vi "DataSimulateModule.vi"(7 "Name(\"\" to use uuid)":string="JKISM-Module") -> ()   [LabVIEW 2014]
uses:
  <userlib>/_NEVSTOP/JKI State Machine++/_Polymophic/Add State(s) to Queue By BOOL(Element).vi
  <userlib>/_NEVSTOP/JKI State Machine++/_Support/JKISMQ/_Obtain JKISMQ.vi
  <userlib>/_NEVSTOP/JKI State Machine++/_Support/FGV-BroadcastRegistry/Cache-Broadcast Registry Search Result.vi
  <userlib>/_NEVSTOP/JKI State Machine++/_Support/JKISMQ/_Create Resp Queue.vi
  <userlib>/_NEVSTOP/JKI State Machine++/_Support/JKISMQ/_Unlock JKISMQ.vi
  <userlib>/_NEVSTOP/JKI State Machine++/_Support/JKISMQ/_Lock State JKISMQ.vi
  <userlib>/_NEVSTOP/JKI State Machine++/_Support/JKISMQ/_Release JKISMQ.vi
  <userlib>/_NEVSTOP/JKI State Machine++/_Support/JKISMQ/_Input Name to JKISM Mode.vi
  <userlib>/_NEVSTOP/JKI State Machine++/Utility/uuid.vi
  <userlib>/_NEVSTOP/JKI State Machine++/_Support/FGV-BroadcastRegistry/global-JKISMQ FGV Change Flag.vi
  <userlib>/_NEVSTOP/JKI State Machine++/_Support/JKISMQ/_JKISMQFGV.vi
  <userlib>/_NEVSTOP/JKI State Machine++/_Support/GlobalEvent/FGV-GlobalEventRef.vi
  <userlib>/_NEVSTOP/JKI State Machine++/_Support/JKISMQ/_Dequeue JKISMQ.vi
  <userlib>/_NEVSTOP/JKI State Machine++/_Support/JKISMQ/_Enqueue JKISMQ.vi
  <userlib>/_NEVSTOP/JKI State Machine++/_Support/FGV-BroadcastRegistry/global-Broadcast Cache Change Flag.vi
  <userlib>/_NEVSTOP/JKI State Machine++/_Support/FGV-BroadcastRegistry/FGV-BroadcastRegistry.vi
  Array-Parameter/_support/FGV-MassData.vi
  Array-Parameter/JKISM++ Array Parameter Support.lvlib
panel:
  out "Error Occurred":errorcluster
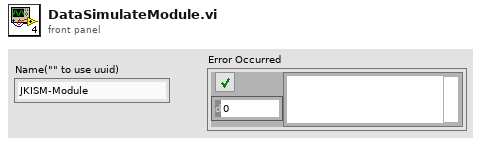
[diagram p1: front panel]
types:
  T1 = enum32{"Invalid", "Standard", "Closed", "Hidden", "Minimized", "Maximized"}
  T2 = enum32{"invalid app kind", "Development System", "Run Time System", "Student Edition", "Embedded LabVIEW", "Evaluation", "Custom"}
  T3 = cluster{"Core":cluster{"Current VI Reference":refnum<vi>, "Close Panel on Exit?":bool}, "DataGen?":bool, "DataSize":i32}
  T4 = cluster{"Current VI Reference":refnum<vi>, "Close Panel on Exit?":bool}
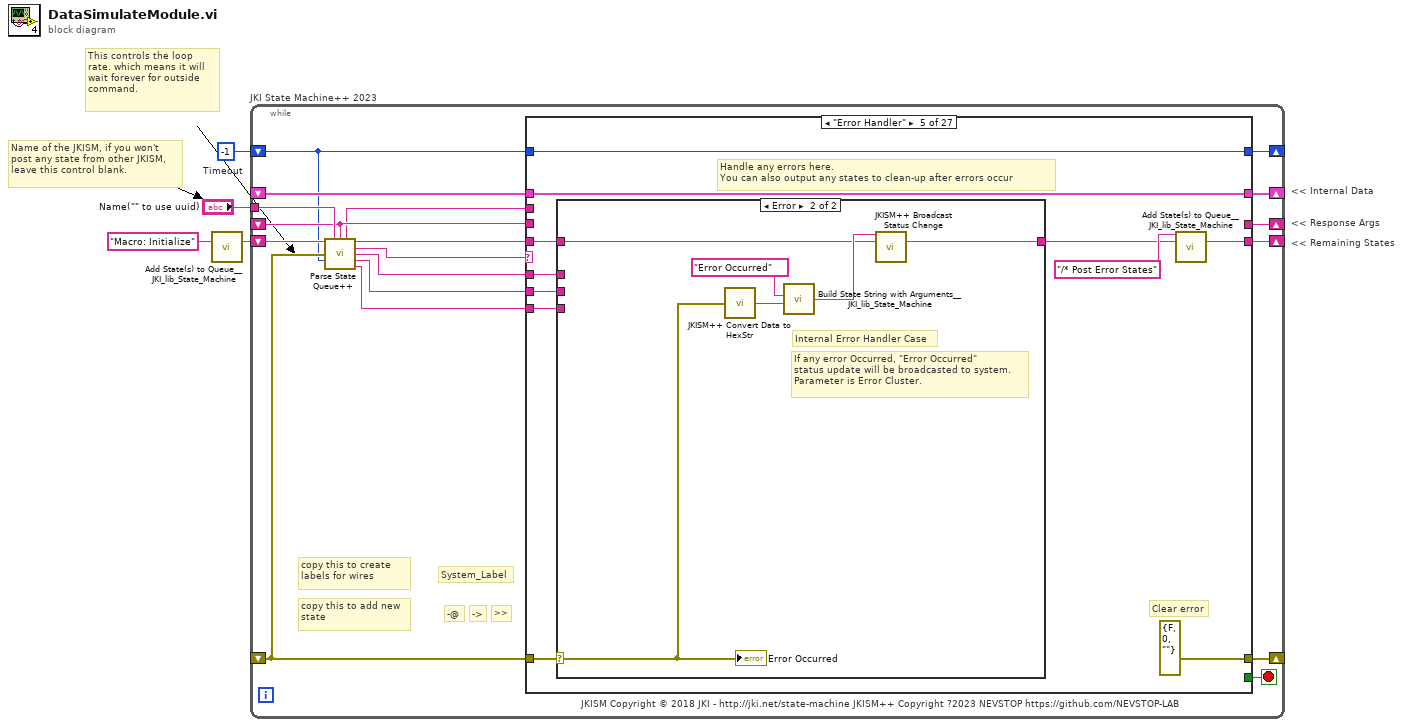
[diagram p0: block diagram]
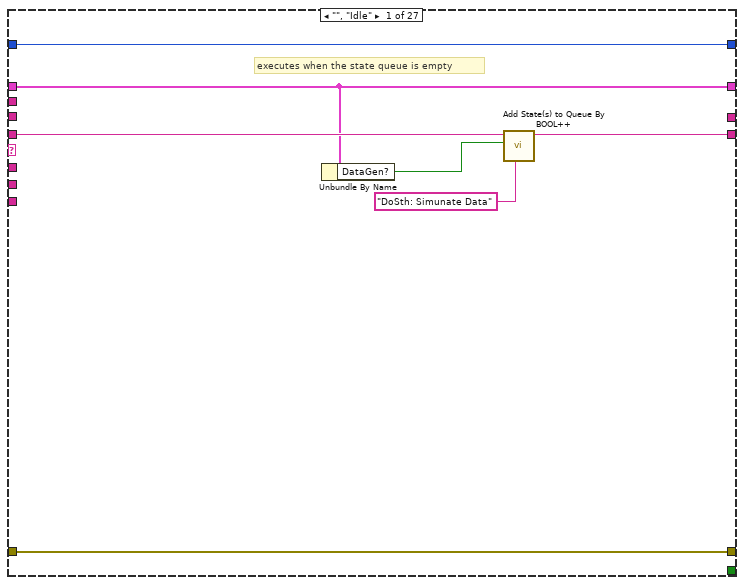
[diagram p2: hidden frame]
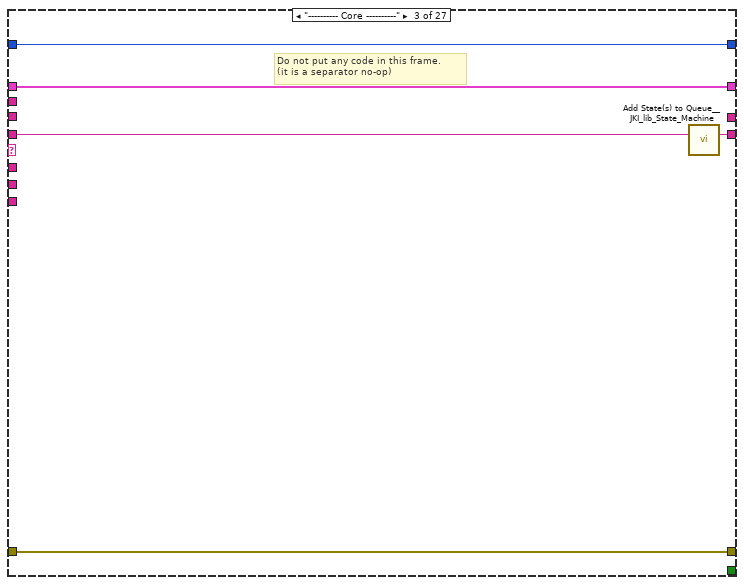
[diagram p4: hidden frame]
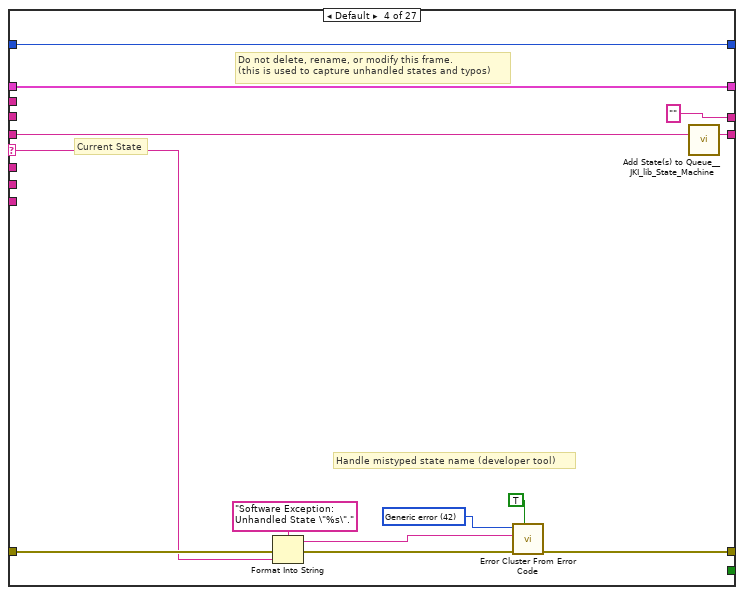
[diagram p5: hidden frame]
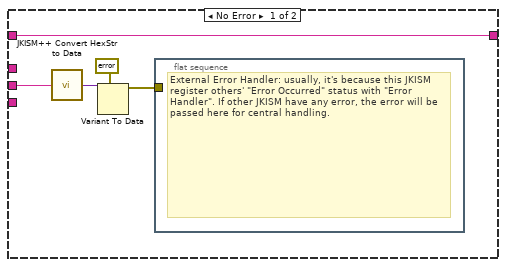
[diagram p6: hidden frame]
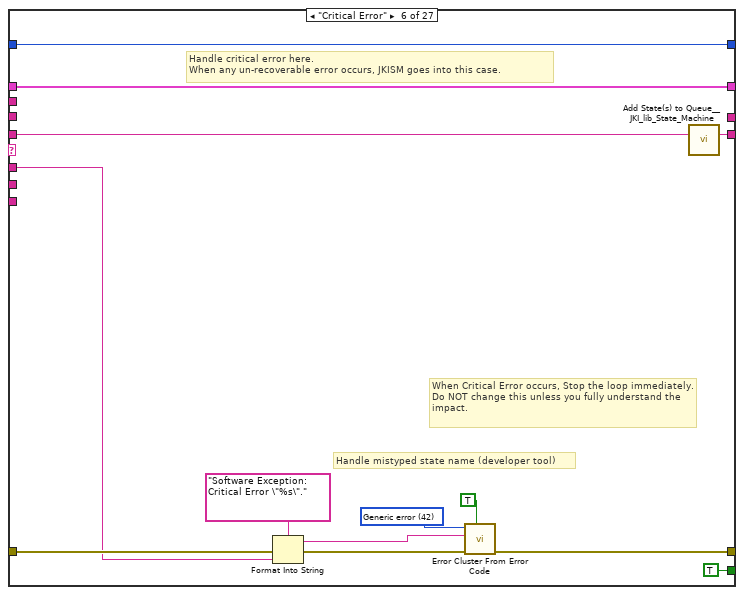
[diagram p7: hidden frame]
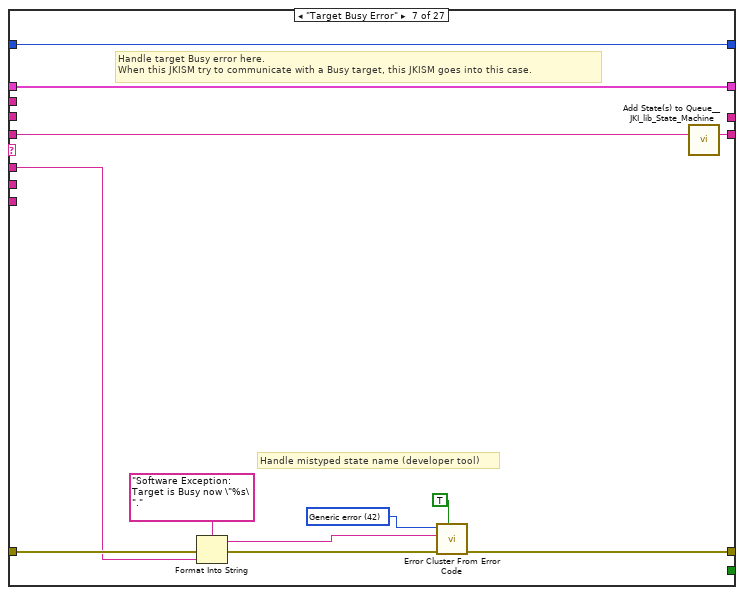
[diagram p8: hidden frame]
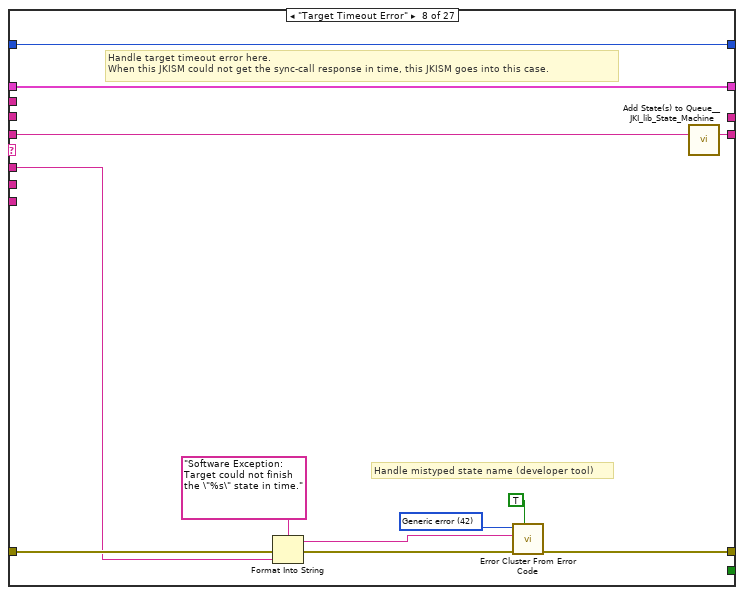
[diagram p9: hidden frame]
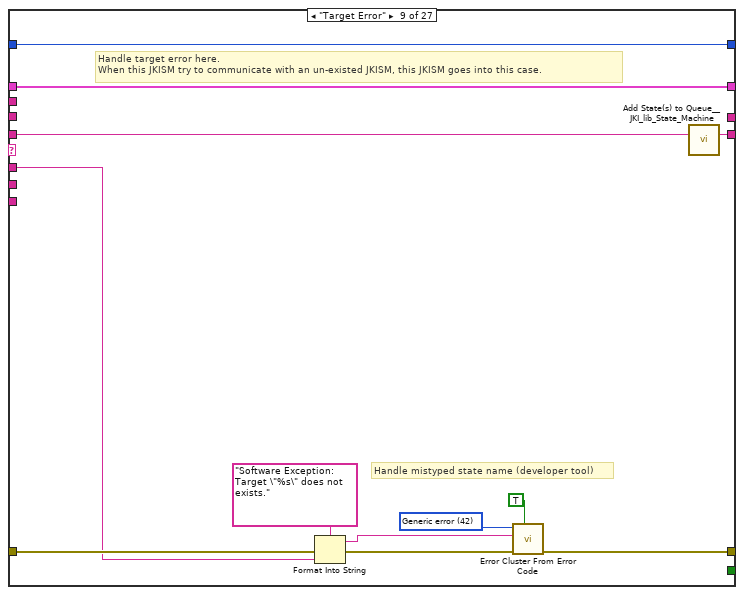
[diagram p10: hidden frame]
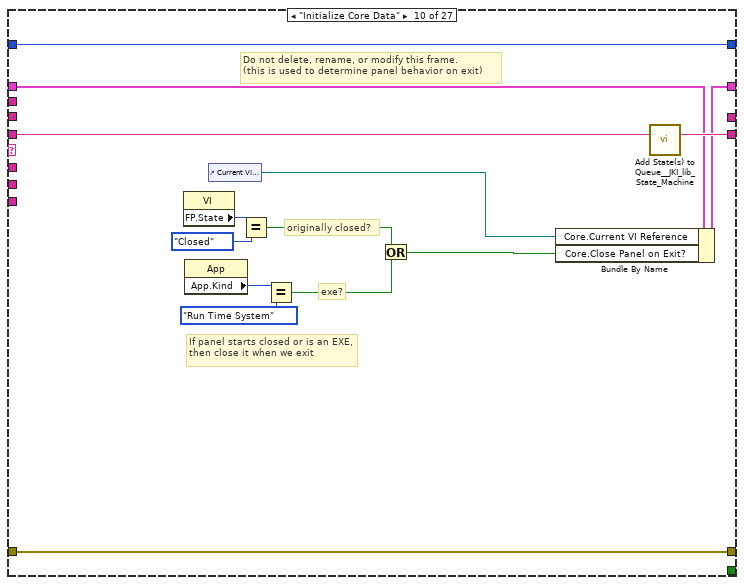
[diagram p11: hidden frame]
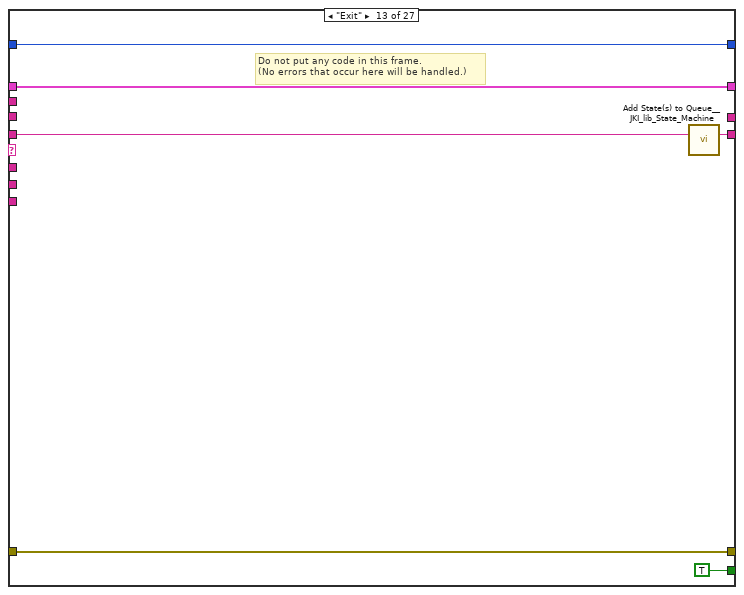
[diagram p14: hidden frame]
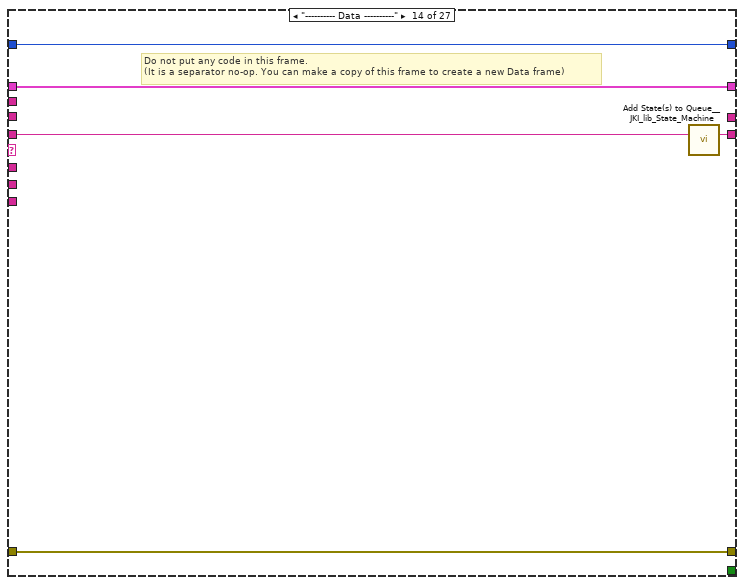
[diagram p15: hidden frame]
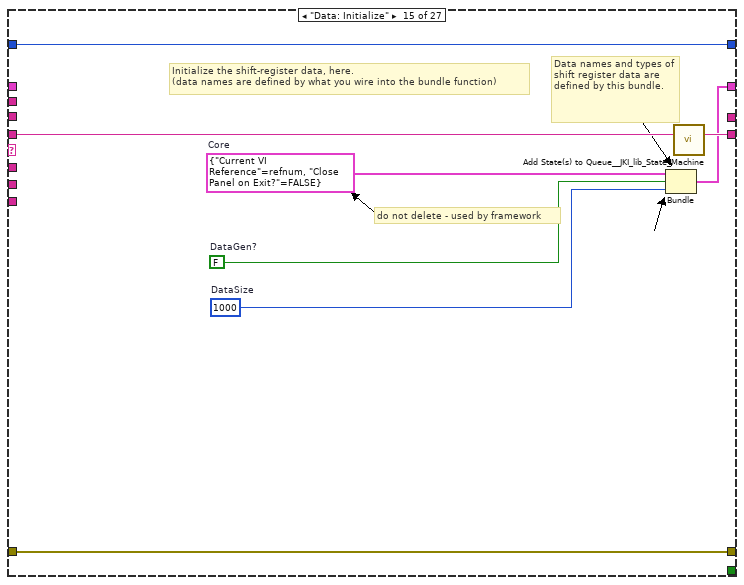
[diagram p16: hidden frame]
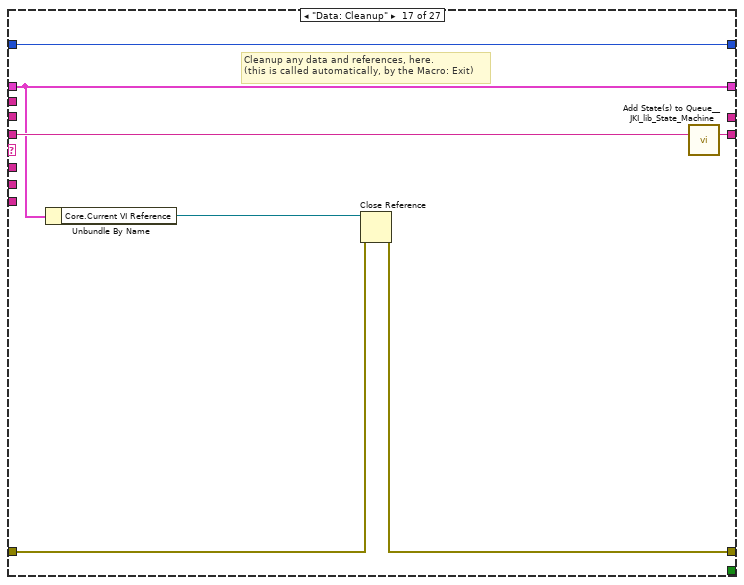
[diagram p18: hidden frame]
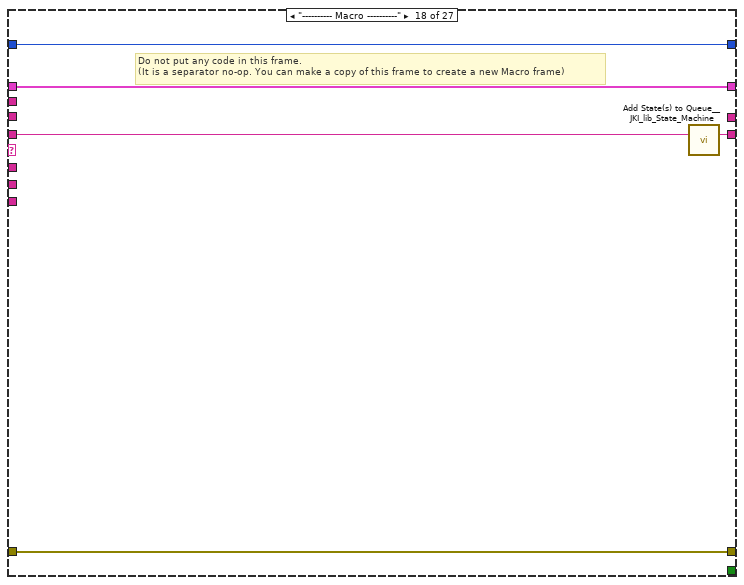
[diagram p19: hidden frame]
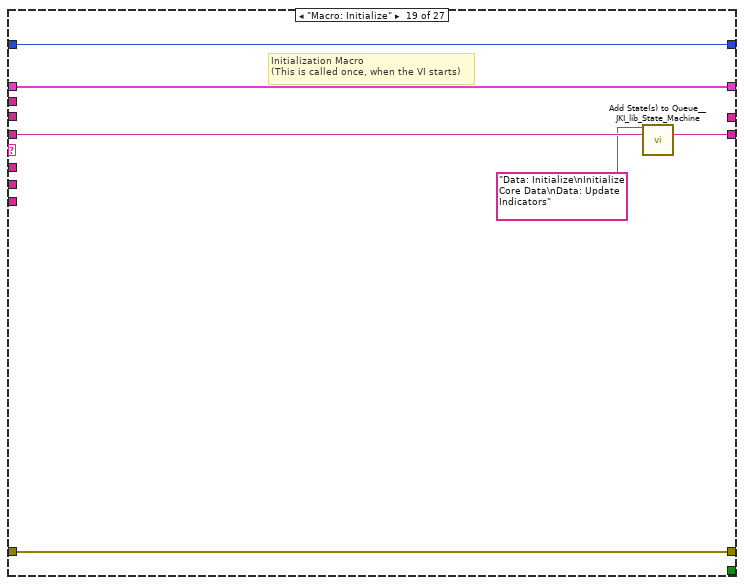
[diagram p20: hidden frame]
diagram:
  w1 = -1  # Timeout
  # "<< Internal Data"
  # "<< Response Args"
  # "<< Remaining States"
  # "Name of the JKISM, if you won't post any state from other JKISM,  leave this control blank."
  # "This controls the loop rate. which means it will wait forever for outside  command."
  n1 = call <vilib>:"Add State(s) to Queue__JKI_lib_State_Machine.vi"("State(s) in (\"\")"="Macro: Initialize") -> ("States Out"=w2:string)  [unwired: 14 in]
  n2 = while "JKI State Machine++ 2023" {
    shift-right: [w17] -> _
    shift-left: _ -> [w16]
    shift-right: [w20] -> _
    shift-left: _ -> [w15]
    shift-right: [w19] -> _
    shift-left: w2 -> [w21]
    tunnel: "Name(\"\" to use uuid)" -> [w13]
    shift-right: [w14] -> _
    shift-left: _ -> [w8]
    shift-right: [w6] -> _
    shift-left: w1 -> [w5]
    stop <- w18 stop-if-true
    # "JKISM Copyright © 2018 JKI - http://jki.net/state-machine JKISM++ Copyright ?2023 NEVSTOP https://github.com/NEVSTOP-LAB"
    # ">>"
    # "copy this to add new state"
    # "->"
    # "-@"
    # "copy this to create labels for wires"
    # "System_Label"
    n3 = call <userlib>:"Parse State Queue++.vi"("State Queue"=w21, "Name(\"\" to use uuid)"=w13, "Response Arguments"=w8, "Error In (no error)"=w15, "Dequeue Timeout(0ms)"=w5) -> ("Name Used"=w7:string, "Remaining States"=w22:string, "Current State"=w9:string, "Arguments"=w10:string, "Argument - State"=w11:string, "From Who"=w12:string)  [unwired: 5 in]
    n4 = case shown="\"Error Handler\"" w9 {
      selector: w9 -> [_ _ _ w41 _ _ _ _ _ _ _ _ _ _ _ _ _ _ _ _ _ _ _ _ _ _ _]
      tunnel: w22 -> [w27 w32 w38 w45 w56 w80 w93 w105 w117 w136 w139 w143 w150 w155 w163 w166 w174 w179 w185 w191 w194 w200 w207 w213 w219 w225 w238]
      tunnel: w10 -> [_ _ _ _ w55 w76 w89 w101 w113 _ _ _ _ _ _ _ _ _ _ _ _ _ w203 _ _ _ _]
      tunnel: w16 -> [w26 w31 w35 w43 w61 w78 w91 w103 w115 w129 w138 w142 w148 w152 _ w165 w169 w176 w182 w188 w193 w199 w206 w212 w218 w222 w232]
      tunnel: [w29 w33 w36 w47 errorcluster {"status"=FALSE, "code"=0, "source"=""} ("error out") w82 w88 w100 w112 w133 w140 w144 w147 w153 w160 w167 w170 w177 w183 w189 w195 w201 w208 w214 w220 w223 w236] -> w20
      tunnel: w15 -> [w29 w33 w36 w46 w59 w81 w94 w106 w118 w133 w140 w144 w147 w153 w160 w167 w171 w177 w183 w189 w195 w201 w208 w214 w220 w223 w236]
      tunnel: [w28 w32 w37 w44 w57 w79 w92 w104 w116 w135 w139 w143 w149 w154 w162 w166 w173 w178 w184 w190 w194 w200 w207 w213 w219 w224 w237] -> w19
      tunnel: [_ _ _ _ _ TRUE _ _ _ _ _ _ TRUE _ _ _ _ _ _ _ _ _ _ _ _ _ _] -> w18
      tunnel: [w26 w31 w35 w43 w61 w78 w91 w103 w115 w134 w138 w142 w148 w152 w161 w165 w169 w176 w182 w188 w193 w198 w205 w212 w217 w222 w232] -> w17
      tunnel: w12 -> [_ _ _ _ w54 _ _ _ _ _ _ _ _ _ _ _ _ _ _ _ _ _ _ _ _ _ _]
      tunnel: w11 -> [_ _ _ _ w53 _ _ _ _ _ _ _ _ _ _ _ _ _ _ _ _ _ _ _ _ _ _]
      tunnel: [_ _ _ "" _ _ _ _ _ _ _ _ _ _ _ _ _ _ _ _ _ _ _ w210 _ _ _] -> w14
      tunnel: w7 -> [_ _ _ _ _ _ _ _ _ _ _ _ _ _ _ _ _ _ _ _ _ _ _ _ _ _ _]
      tunnel: w8 -> [_ _ _ _ _ _ _ _ _ _ _ _ _ _ _ _ _ _ _ _ _ _ _ _ _ _ _]
      tunnel: [w23 w30 w34 w39 w52 w74 w87 w99 w111 w123 w137 w141 w145 w151 w156 w164 w168 w175 w180 w186 w192 200 ("Timeout") w202 w209 -1 ("Timeout") w221 w229] -> w6
      tunnel: w5 -> [w23 w30 w34 w39 w52 w74 w87 w99 w111 w123 w137 w141 w145 w151 w156 w164 w168 w175 w180 w186 w192 _ w202 w209 _ w221 w229]
      frame "", "Idle" {
        # "executes when the state queue is empty"
        n5 = Unbundle By Name(w26) -> ("DataGen?"=w25:bool)
        n6 = call-poly <userlib>:"Add State(s) to Queue By BOOL++.vi"("TRUE(\"\")"="DoSth: Simunate Data" ("TRUE(\"\")"), "Bool"=w25, "State Queue(\"\")"=w27) -> ("State Queue Out"=w28:string)  [unwired: 8 in]
      }
      frame "JKISM++ Documentation" {
        # "JKISM++ Documentation"
        # "State Syntax:\nStateCategory: State >> Argument -@ JKISMName\nStateCategory: State >> Argument -> JKISMName\n\nLine Terminator: Line feed"
        # "Commenting:\nTo add a comment use \"//\" or \"#\" and all text to the right will be ignored\nCommenting Example:\nUI: Initialize // This initializes the UI\n// Another comment line"
        # "Example:\nUI: Help >> About -@Main\nUI: Help >> About ->Main\n\nWhere \"UI\" is the state category\nWhere \"Help\" is the state\nWhere \"About\" is the argument\nWhere \"Main\" is the Name of JKISM,which actually run the \"UI: Help >> About\"\n\n    \"-@\" stands for sync state. Current JKISM will wait until the state is finished. \n            - if \"Main\" named JKISM does not exist, \"Target Error\" will occur.\n            - if \"Main\" named JKISM is in another sync remote state, \"Target Busy Error\" will occur.\n            - if \"Main\" named JKISM could not finish the state in time, \"Target Timeout Error\" will occur.\n            - if everything is right. \"Response\" will occur with Argument back from \"Main\" named JKISM. \n\n    \"->\" stands for async state. Current JKISM will post the state and continue to next state in next iteration.\n            - if \"Main\" named JKISM does not exist, \"Target Error\" will occur.\n            - if everything is right. \"Async Message Posted\" will occur.\n            - After State is finished. Caller will receive a \"Async Response\" state from callee.\n\nWhen duplicated name is used for multiple JKISM module or some framework problem happens, \"Critical Error\" will occur."
      }
      frame "---------- Core ----------" {
        # "Do not put any code in this frame.\n(it is a separator no-op)"
        n7 = call <vilib>:"Add State(s) to Queue__JKI_lib_State_Machine.vi"("State(s) in (\"\")"=w38) -> ("States Out"=w37:string)  [unwired: 14 in]
      }
      frame Default {
        w50 = 42 items=["No error", "Argument error", "Memory is full", "Out of zone", "End of file", "File already open", "Generic file I/O error", "File not found", "File permission error", "Disk is full", "Duplicate path", "Too many files open", "System feature not enabled", "Resource file not found", "Cannot add resource", "Resource not found", "Image not found", "Image memory error", "Pen does not exist", "Config type invalid", "Config token not found", "Config parse error", "Config memory error", "Bad external code format", "Bad external code offset", "External code not present", "Null window", "Destroy window error", "Null menu", "Print aborted", "Bad print record", "Print driver error", "Windows error during printing", "Memory error during printing", "Print dialog error", "Generic print error", "Invalid device refnum", "Device not found", "Device parameter error", "Device unit error", "Cannot open device", "Device call aborted", "Generic error", "Cancelled by user", "Object ID too low", "Object ID too high", "Object not in heap", "Unknown heap", "Unknown object (invalid DefProc)", "Unknown object (DefProc not in table)", "Message out of range", "Invalid (null) method", "Unknown message", "Manager call not supported", "Bad address", "Network operation in progress", "Network operation timed out", "Connection is busy", "Network attribute not supported", "Network error", "Address in use", "System out of memory", "Connection aborted", "Connection refused", "Not connected", "Already connected", "Connection closed", "Initialization error (interapplication manager)", "Bad occurrence", "Wait on unbound occurrence handler", "Occurrence queue overflow", "Datalog type conflict", "Unused", "Unrecognized type (interapplication manager)", "Memory corrupt", "Failed to make temporary DLL", "Old CIN version", "Drag socket not found", "Failed to load drop-object", "Failed to register OLE object", "Failed to release OLE object", "Format specifier type mismatch", "Unknown format specifier", "Too few format specifiers", "Too many format specifiers", "Scan failed", "Newer CIN version", "Error converting to variant", "Runtime menu error", "Password tampered", "Variant attribute not found", "Incompatible variant data type", "Event data is not available", "Event Store is not present", "Occurrence is not found", "Event Queue is not created", "Event info is not available", "Refnum passed is NULL", "Error retrieving Class GUID", "Error retrieving CoClass GUID", "Error retrieving TypeLib GUID.", "Bad built application magic bytes.", "Specific driver is different from the specific driver associated with the Logical Name.", "There is no session opened to the class driver.", "Max Error", "MAX - Error with config objects", "MAX - Error loading configuration", "MAX - Group not supported"]
        # "Current State"
        # "Do not delete, rename, or modify this frame.\n(this is used to capture unhandled states and typos)"
        # "Handle mistyped state name (developer tool)"
        n8 = Format Into String(format string="Software Exception: Unhandled State \"%s\"." ("message"), error in=w46, w41) -> (resulting string=w49:string, error out=w48:errorcluster)  [unwired: 1 in]
        n9 = call <vilib>:"Error Cluster From Error Code.vi"("show call chain? (False)"=TRUE, "error in (no error)"=w48, "error message (\"\")"=w49, "error code (0)"=w50) -> ("error out"=w47:errorcluster)  [unwired: 5 in]
        n10 = call <vilib>:"Add State(s) to Queue__JKI_lib_State_Machine.vi"("State(s) in (\"\")"=w45) -> ("States Out"=w44:string)  [unwired: 14 in]
      }
      frame "Error Handler" {
        # "Handle any errors here.\nYou can also output any states to clean-up after errors occur"
        # "Clear error"
        n11 = case shown="Error" w59 {
          selector: w59 -> [_ w71]
          tunnel: [w67 w69] -> w58
          tunnel: w56 -> [w67 w68]
          tunnel: w55 -> [_ _]
          tunnel: w54 -> [_ _]
          tunnel: w53 -> [w66 _]
          frame No Error {
            n12 = call <userlib>:"JKISM++ Convert HexStr to Data.vi"("HEX String"=w66) -> ("Variant"=w65:variant)  [unwired: 8 in]
            n13 = Variant To Data(type=errorcluster {"status"=FALSE, "code"=0, "source"=""} ("error in (no error)"), Variant=w65) -> (data=w63:errorcluster)  [unwired: 1 in, 1 out]
            n14 = flat-sequence {
              tunnel: w63 -> [_]
              frame #0 {
                # "External Error Handler: usually, it's because this JKISM register others' \"Error Occurred\" status with \"Error Handler\". If other JKISM have any error, the error will be passed here for central handling."
              }
            }
          }
          frame Error {
            # "Internal Error Handler Case"
            # "If any error Occurred, \"Error Occurred\" \nstatus update will be broadcasted to system.\nParameter is Error Cluster."
            n15 = call <userlib>:"JKISM++ Convert Data to HexStr.vi"("Variant"=w71) -> ("HEX String (0-9,A-F)"=w72:string)  [unwired: 8 in]
            n16 = call <vilib>:"Build State String with Arguments__JKI_lib_State_Machine.vi"("Arguments (\"\")"=w72, "State"="Error Occurred" ("Status with Arguments")) -> ("State with Arguments"=w70:string)  [unwired: 4 in]
            n17 = call <userlib>:"JKISM++ Broadcast Status Change.vi"("Status with Arguments"=w70, "State Queue"=w68) -> ("Remaining States"=w69:string)  [unwired: 13 in]
            "Error Occurred" <- w71
          }
        }
        n18 = call <vilib>:"Add State(s) to Queue__JKI_lib_State_Machine.vi"("State(s) in Front (\"\")"="/* Post Error States", "State(s) in (\"\")"=w58) -> ("States Out"=w57:string)  [unwired: 13 in]
      }
      frame "Critical Error" {
        w85 = 42 items=["No error", "Argument error", "Memory is full", "Out of zone", "End of file", "File already open", "Generic file I/O error", "File not found", "File permission error", "Disk is full", "Duplicate path", "Too many files open", "System feature not enabled", "Resource file not found", "Cannot add resource", "Resource not found", "Image not found", "Image memory error", "Pen does not exist", "Config type invalid", "Config token not found", "Config parse error", "Config memory error", "Bad external code format", "Bad external code offset", "External code not present", "Null window", "Destroy window error", "Null menu", "Print aborted", "Bad print record", "Print driver error", "Windows error during printing", "Memory error during printing", "Print dialog error", "Generic print error", "Invalid device refnum", "Device not found", "Device parameter error", "Device unit error", "Cannot open device", "Device call aborted", "Generic error", "Cancelled by user", "Object ID too low", "Object ID too high", "Object not in heap", "Unknown heap", "Unknown object (invalid DefProc)", "Unknown object (DefProc not in table)", "Message out of range", "Invalid (null) method", "Unknown message", "Manager call not supported", "Bad address", "Network operation in progress", "Network operation timed out", "Connection is busy", "Network attribute not supported", "Network error", "Address in use", "System out of memory", "Connection aborted", "Connection refused", "Not connected", "Already connected", "Connection closed", "Initialization error (interapplication manager)", "Bad occurrence", "Wait on unbound occurrence handler", "Occurrence queue overflow", "Datalog type conflict", "Unused", "Unrecognized type (interapplication manager)", "Memory corrupt", "Failed to make temporary DLL", "Old CIN version", "Drag socket not found", "Failed to load drop-object", "Failed to register OLE object", "Failed to release OLE object", "Format specifier type mismatch", "Unknown format specifier", "Too few format specifiers", "Too many format specifiers", "Scan failed", "Newer CIN version", "Error converting to variant", "Runtime menu error", "Password tampered", "Variant attribute not found", "Incompatible variant data type", "Event data is not available", "Event Store is not present", "Occurrence is not found", "Event Queue is not created", "Event info is not available", "Refnum passed is NULL", "Error retrieving Class GUID", "Error retrieving CoClass GUID", "Error retrieving TypeLib GUID.", "Bad built application magic bytes.", "Specific driver is different from the specific driver associated with the Logical Name.", "There is no session opened to the class driver.", "Max Error", "MAX - Error with config objects", "MAX - Error loading configuration", "MAX - Group not supported"]
        # "Handle critical error here.\nWhen any un-recoverable error occurs, JKISM goes into this case."
        # "When Critical Error occurs, Stop the loop immediately. Do NOT change this unless you fully understand the impact."
        # "Handle mistyped state name (developer tool)"
        n19 = Format Into String(format string="Software Exception: Critical Error \"%s\"." ("message"), error in=w81, w76) -> (resulting string=w84:string, error out=w83:errorcluster)  [unwired: 1 in]
        n20 = call <vilib>:"Error Cluster From Error Code.vi"("show call chain? (False)"=TRUE, "error in (no error)"=w83, "error message (\"\")"=w84, "error code (0)"=w85) -> ("error out"=w82:errorcluster)  [unwired: 5 in]
        n21 = call <vilib>:"Add State(s) to Queue__JKI_lib_State_Machine.vi"("State(s) in (\"\")"=w80) -> ("States Out"=w79:string)  [unwired: 14 in]
      }
      frame "Target Busy Error" {
        w97 = 42 items=["No error", "Argument error", "Memory is full", "Out of zone", "End of file", "File already open", "Generic file I/O error", "File not found", "File permission error", "Disk is full", "Duplicate path", "Too many files open", "System feature not enabled", "Resource file not found", "Cannot add resource", "Resource not found", "Image not found", "Image memory error", "Pen does not exist", "Config type invalid", "Config token not found", "Config parse error", "Config memory error", "Bad external code format", "Bad external code offset", "External code not present", "Null window", "Destroy window error", "Null menu", "Print aborted", "Bad print record", "Print driver error", "Windows error during printing", "Memory error during printing", "Print dialog error", "Generic print error", "Invalid device refnum", "Device not found", "Device parameter error", "Device unit error", "Cannot open device", "Device call aborted", "Generic error", "Cancelled by user", "Object ID too low", "Object ID too high", "Object not in heap", "Unknown heap", "Unknown object (invalid DefProc)", "Unknown object (DefProc not in table)", "Message out of range", "Invalid (null) method", "Unknown message", "Manager call not supported", "Bad address", "Network operation in progress", "Network operation timed out", "Connection is busy", "Network attribute not supported", "Network error", "Address in use", "System out of memory", "Connection aborted", "Connection refused", "Not connected", "Already connected", "Connection closed", "Initialization error (interapplication manager)", "Bad occurrence", "Wait on unbound occurrence handler", "Occurrence queue overflow", "Datalog type conflict", "Unused", "Unrecognized type (interapplication manager)", "Memory corrupt", "Failed to make temporary DLL", "Old CIN version", "Drag socket not found", "Failed to load drop-object", "Failed to register OLE object", "Failed to release OLE object", "Format specifier type mismatch", "Unknown format specifier", "Too few format specifiers", "Too many format specifiers", "Scan failed", "Newer CIN version", "Error converting to variant", "Runtime menu error", "Password tampered", "Variant attribute not found", "Incompatible variant data type", "Event data is not available", "Event Store is not present", "Occurrence is not found", "Event Queue is not created", "Event info is not available", "Refnum passed is NULL", "Error retrieving Class GUID", "Error retrieving CoClass GUID", "Error retrieving TypeLib GUID.", "Bad built application magic bytes.", "Specific driver is different from the specific driver associated with the Logical Name.", "There is no session opened to the class driver.", "Max Error", "MAX - Error with config objects", "MAX - Error loading configuration", "MAX - Group not supported"]
        # "Handle target Busy error here.\nWhen this JKISM try to communicate with a Busy target, this JKISM goes into this case."
        # "Handle mistyped state name (developer tool)"
        n22 = Format Into String(format string="Software Exception: Target is Busy now \"%s\"." ("message"), error in=w94, w89) -> (resulting string=w96:string, error out=w95:errorcluster)  [unwired: 1 in]
        n23 = call <vilib>:"Error Cluster From Error Code.vi"("show call chain? (False)"=TRUE, "error in (no error)"=w95, "error message (\"\")"=w96, "error code (0)"=w97) -> ("error out"=w88:errorcluster)  [unwired: 5 in]
        n24 = call <vilib>:"Add State(s) to Queue__JKI_lib_State_Machine.vi"("State(s) in (\"\")"=w93) -> ("States Out"=w92:string)  [unwired: 14 in]
      }
      frame "Target Timeout Error" {
        w109 = 42 items=["No error", "Argument error", "Memory is full", "Out of zone", "End of file", "File already open", "Generic file I/O error", "File not found", "File permission error", "Disk is full", "Duplicate path", "Too many files open", "System feature not enabled", "Resource file not found", "Cannot add resource", "Resource not found", "Image not found", "Image memory error", "Pen does not exist", "Config type invalid", "Config token not found", "Config parse error", "Config memory error", "Bad external code format", "Bad external code offset", "External code not present", "Null window", "Destroy window error", "Null menu", "Print aborted", "Bad print record", "Print driver error", "Windows error during printing", "Memory error during printing", "Print dialog error", "Generic print error", "Invalid device refnum", "Device not found", "Device parameter error", "Device unit error", "Cannot open device", "Device call aborted", "Generic error", "Cancelled by user", "Object ID too low", "Object ID too high", "Object not in heap", "Unknown heap", "Unknown object (invalid DefProc)", "Unknown object (DefProc not in table)", "Message out of range", "Invalid (null) method", "Unknown message", "Manager call not supported", "Bad address", "Network operation in progress", "Network operation timed out", "Connection is busy", "Network attribute not supported", "Network error", "Address in use", "System out of memory", "Connection aborted", "Connection refused", "Not connected", "Already connected", "Connection closed", "Initialization error (interapplication manager)", "Bad occurrence", "Wait on unbound occurrence handler", "Occurrence queue overflow", "Datalog type conflict", "Unused", "Unrecognized type (interapplication manager)", "Memory corrupt", "Failed to make temporary DLL", "Old CIN version", "Drag socket not found", "Failed to load drop-object", "Failed to register OLE object", "Failed to release OLE object", "Format specifier type mismatch", "Unknown format specifier", "Too few format specifiers", "Too many format specifiers", "Scan failed", "Newer CIN version", "Error converting to variant", "Runtime menu error", "Password tampered", "Variant attribute not found", "Incompatible variant data type", "Event data is not available", "Event Store is not present", "Occurrence is not found", "Event Queue is not created", "Event info is not available", "Refnum passed is NULL", "Error retrieving Class GUID", "Error retrieving CoClass GUID", "Error retrieving TypeLib GUID.", "Bad built application magic bytes.", "Specific driver is different from the specific driver associated with the Logical Name.", "There is no session opened to the class driver.", "Max Error", "MAX - Error with config objects", "MAX - Error loading configuration", "MAX - Group not supported"]
        # "Handle target timeout error here.\nWhen this JKISM could not get the sync-call response in time, this JKISM goes into this case."
        # "Handle mistyped state name (developer tool)"
        n25 = Format Into String(format string="Software Exception: Target could not finish the \"%s\" state in time." ("message"), error in=w106, w101) -> (resulting string=w108:string, error out=w107:errorcluster)  [unwired: 1 in]
        n26 = call <vilib>:"Error Cluster From Error Code.vi"("show call chain? (False)"=TRUE, "error in (no error)"=w107, "error message (\"\")"=w108, "error code (0)"=w109) -> ("error out"=w100:errorcluster)  [unwired: 5 in]
        n27 = call <vilib>:"Add State(s) to Queue__JKI_lib_State_Machine.vi"("State(s) in (\"\")"=w105) -> ("States Out"=w104:string)  [unwired: 14 in]
      }
      frame "Target Error" {
        w121 = 42 items=["No error", "Argument error", "Memory is full", "Out of zone", "End of file", "File already open", "Generic file I/O error", "File not found", "File permission error", "Disk is full", "Duplicate path", "Too many files open", "System feature not enabled", "Resource file not found", "Cannot add resource", "Resource not found", "Image not found", "Image memory error", "Pen does not exist", "Config type invalid", "Config token not found", "Config parse error", "Config memory error", "Bad external code format", "Bad external code offset", "External code not present", "Null window", "Destroy window error", "Null menu", "Print aborted", "Bad print record", "Print driver error", "Windows error during printing", "Memory error during printing", "Print dialog error", "Generic print error", "Invalid device refnum", "Device not found", "Device parameter error", "Device unit error", "Cannot open device", "Device call aborted", "Generic error", "Cancelled by user", "Object ID too low", "Object ID too high", "Object not in heap", "Unknown heap", "Unknown object (invalid DefProc)", "Unknown object (DefProc not in table)", "Message out of range", "Invalid (null) method", "Unknown message", "Manager call not supported", "Bad address", "Network operation in progress", "Network operation timed out", "Connection is busy", "Network attribute not supported", "Network error", "Address in use", "System out of memory", "Connection aborted", "Connection refused", "Not connected", "Already connected", "Connection closed", "Initialization error (interapplication manager)", "Bad occurrence", "Wait on unbound occurrence handler", "Occurrence queue overflow", "Datalog type conflict", "Unused", "Unrecognized type (interapplication manager)", "Memory corrupt", "Failed to make temporary DLL", "Old CIN version", "Drag socket not found", "Failed to load drop-object", "Failed to register OLE object", "Failed to release OLE object", "Format specifier type mismatch", "Unknown format specifier", "Too few format specifiers", "Too many format specifiers", "Scan failed", "Newer CIN version", "Error converting to variant", "Runtime menu error", "Password tampered", "Variant attribute not found", "Incompatible variant data type", "Event data is not available", "Event Store is not present", "Occurrence is not found", "Event Queue is not created", "Event info is not available", "Refnum passed is NULL", "Error retrieving Class GUID", "Error retrieving CoClass GUID", "Error retrieving TypeLib GUID.", "Bad built application magic bytes.", "Specific driver is different from the specific driver associated with the Logical Name.", "There is no session opened to the class driver.", "Max Error", "MAX - Error with config objects", "MAX - Error loading configuration", "MAX - Group not supported"]
        # "Handle target error here.\nWhen this JKISM try to communicate with an un-existed JKISM, this JKISM goes into this case."
        # "Handle mistyped state name (developer tool)"
        n28 = Format Into String(format string="Software Exception: Target \"%s\" does not exists." ("message"), error in=w118, w113) -> (resulting string=w120:string, error out=w119:errorcluster)  [unwired: 1 in]
        n29 = call <vilib>:"Error Cluster From Error Code.vi"("show call chain? (False)"=TRUE, "error in (no error)"=w119, "error message (\"\")"=w120, "error code (0)"=w121) -> ("error out"=w112:errorcluster)  [unwired: 5 in]
        n30 = call <vilib>:"Add State(s) to Queue__JKI_lib_State_Machine.vi"("State(s) in (\"\")"=w117) -> ("States Out"=w116:string)  [unwired: 14 in]
      }
      frame "Initialize Core Data" {
        # "Do not delete, rename, or modify this frame.\n(this is used to determine panel behavior on exit)"
        # "originally closed?"
        # "exe?"
        # "If panel starts closed or is an EXE, then close it when we exit"
        n31 = property class="VI"() -> ("FP.State"=w126:T1)  [unwired: 2 in, 2 out]
        n32 = property class="App"() -> ("App.Kind"=w132:T2)  [unwired: 2 in, 2 out]
        n33 = control-ref of="Current VI Reference"() -> (w127:refnum<vi>)
        n34 = Equal?(x=w126, y=T1."Closed" ("Front Panel Window:State")) -> (x = y?=w124:bool)
        n35 = Equal?(x=w132, y=T2."Run Time System" ("Application:Kind")) -> (x = y?=w130:bool)
        n36 = Or(x=w124, y=w130) -> (x .or. y?=w128:bool)
        n37 = Bundle By Name(cluster=w129, "Core.Current VI Reference"=w127, "Core.Close Panel on Exit?"=w128) -> (w134:T3)
        n38 = call <vilib>:"Add State(s) to Queue__JKI_lib_State_Machine.vi"("State(s) in (\"\")"=w136) -> ("States Out"=w135:string)  [unwired: 14 in]
      }
      frame "Async Response", "Response" {
      }
      frame "Async Message Posted" {
      }
      frame "Exit" {
        # "Do not put any code in this frame.\n(No errors that occur here will be handled.)"
        n39 = call <vilib>:"Add State(s) to Queue__JKI_lib_State_Machine.vi"("State(s) in (\"\")"=w150) -> ("States Out"=w149:string)  [unwired: 14 in]
      }
      frame "---------- Data ----------" {
        # "Do not put any code in this frame.\n(It is a separator no-op. You can make a copy of this frame to create a new Data frame)"
        n40 = call <vilib>:"Add State(s) to Queue__JKI_lib_State_Machine.vi"("State(s) in (\"\")"=w155) -> ("States Out"=w154:string)  [unwired: 14 in]
      }
      frame "Data: Initialize" {
        w157 = 1000  # DataSize
        w158 = T4 {"Current VI Reference"=refnum, "Close Panel on Exit?"=FALSE}  # Core
        w159 = FALSE  # DataGen?
        # "do not delete - used by framework"
        # "Data names and types of shift register data are defined by this bundle."
        # "Initialize the shift-register data, here.\n(data names are defined by what you wire into the bundle function)"
        n41 = Bundle("Core"=w158, "DataGen?"=w159, "DataSize"=w157) -> (w161:T3)  [unwired: 1 in]
        n42 = call <vilib>:"Add State(s) to Queue__JKI_lib_State_Machine.vi"("State(s) in (\"\")"=w163) -> ("States Out"=w162:string)  [unwired: 14 in]
      }
      frame "Data: Update Indicators" {
      }
      frame "Data: Cleanup" {
        # "Cleanup any data and references, here.\n(this is called automatically, by the Macro: Exit)"
        n43 = Unbundle By Name(w169) -> ("Core.Current VI Reference"=w172:refnum<vi>)
        n44 = Close Reference(reference=w172, error in (no error)=w171) -> (error out=w170:errorcluster)
        n45 = call <vilib>:"Add State(s) to Queue__JKI_lib_State_Machine.vi"("State(s) in (\"\")"=w174) -> ("States Out"=w173:string)  [unwired: 14 in]
      }
      frame "---------- Macro ----------" {
        # "Do not put any code in this frame.\n(It is a separator no-op. You can make a copy of this frame to create a new Macro frame)"
        n46 = call <vilib>:"Add State(s) to Queue__JKI_lib_State_Machine.vi"("State(s) in (\"\")"=w179) -> ("States Out"=w178:string)  [unwired: 14 in]
      }
      frame "Macro: Initialize" {
        # "Initialization Macro\n(This is called once, when the VI starts)"
        n47 = call <vilib>:"Add State(s) to Queue__JKI_lib_State_Machine.vi"("State(s) in Front (\"\")"="Data: Initialize\nInitialize Core Data\nData: Update Indicators", "State(s) in (\"\")"=w185) -> ("States Out"=w184:string)  [unwired: 13 in]
      }
      frame "Macro: Exit" {
        # "Exit Macro\n(This is called once, when the VI exits)"
        n48 = call <vilib>:"Add State(s) to Queue__JKI_lib_State_Machine.vi"("State(s) in Front (\"\")"="Data: Cleanup\nExit", "State(s) in (\"\")"=w191) -> ("States Out"=w190:string)  [unwired: 13 in]
      }
      frame "---------- API ----------" {
        # "Do not put any code in this frame.\n(It is a separator no-op. This category is recommended to use for external API)"
      }
      frame "API: Start" {
        # "Copy/Rename this case for your own API"
        n49 = Bundle By Name(cluster=w199, "DataGen?"=TRUE) -> (w198:T3)
      }
      frame "API: Config Data Size" {
        n50 = Decimal String To Number(string=w203) -> (number=w204:i32)  [unwired: 2 in, 1 out]
        n51 = Bundle By Name(cluster=w206, "DataSize"=w204) -> (w205:T3)
      }
      frame "API: Data Size" {
        n52 = Unbundle By Name(w212) -> ("DataSize"=w211:i32)
        n53 = Format Into String(w211) -> (resulting string=w210:string)  [unwired: 3 in, 1 out]
      }
      frame "API: Stop" {
        # "Copy/Rename this case for your own API"
        n54 = Bundle By Name(cluster=w218, "DataGen?"=FALSE) -> (w217:T3)
      }
      frame "---------- DoSth ----------" {
        # "Template Separator\n(You can make a copy of, or modify, this frame)"
        n55 = call <vilib>:"Add State(s) to Queue__JKI_lib_State_Machine.vi"("State(s) in (\"\")"=w225) -> ("States Out"=w224:string)  [unwired: 14 in]
      }
      frame "DoSth: Simunate Data" {
        # "Your code here.\n(You can make a copy of, or modify, this frame)"
        n56 = Unbundle By Name(w232) -> ("DataSize"=w231:i32)
        n57 = feedback #1(0.01 ("x")) -> (w227:dbl)
        n58 = for {
          N: w231 -> [_]
          tunnel: [w242] -> w230 mode=indexing
          shift-right: [w239] -> w226
          shift-left: w227 -> [w241]
          n59 = Add(x=0.01, y=w241) -> (x+y=w239:dbl)
          n60 = Sine(x=w239) -> (sin(x)=w242:dbl)
        }
        n61 = feedback-in #1(w226) -> ()
        n62 = call "JKISM++ Convert Array to Argument.vi"("DBL"=w230) -> ("Argument"=w235:string)  [unwired: 8 in]
        n63 = call <vilib>:"Build State String with Arguments__JKI_lib_State_Machine.vi"("Arguments (\"\")"=w235, "State"="Simulated Data") -> ("State with Arguments"=w233:string)  [unwired: 4 in]
        n64 = call <userlib>:"JKISM++ Broadcast Status Change.vi"("Status with Arguments"=w233, "State Queue"=w238) -> ("Remaining States"=w237:string)  [unwired: 13 in]
      }
    }
  }
